vi "tb_host transfer.vi"() -> ()   [LabVIEW 2012]
uses:
  <userlib>/FPGA Library/Code Development/DRAM/2 Bank DRAM/Data Type (256).ctl
  <vilib>/Platform/TimedLoop/XDataNode/timing_clust.ctl
  <vilib>/Platform/TimedLoop/XDataNode/nitl_modes.ctl
  <vilib>/Platform/TimedLoop/XDataNode/wakeup.ctl
  <vilib>/rvi/Emulation/niFpgaSctlEmulationRegisterWithScheduler.vi
  <vilib>/rvi/Emulation/niFpgaSctlEmulationScheduler.vi
  <vilib>/platform/TimedLoop/XDataNode/XDataNode.xnode
  <vilib>/Platform/TimedLoop/XDataNode/XDNodeRunTimeDep.lvlib
panel:
  in  "stop":bool
  out "Data into FIFO":u64[](array[numeric])
  out "Input Data":T1
  out "Data to FIFO":u64(graph)
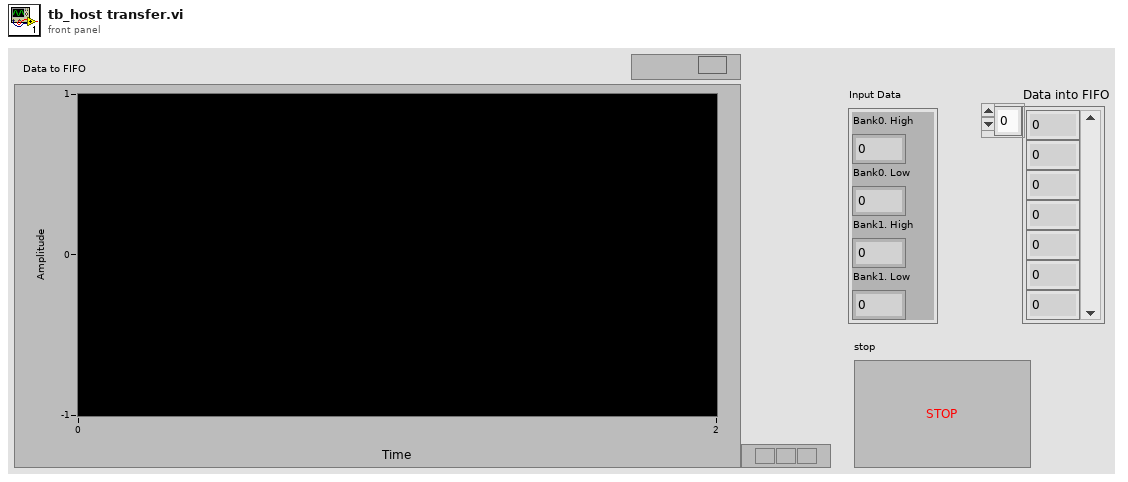
[diagram p1: front panel]
types:
  T1 = typedef "Data Type (256).ctl" = cluster{"Bank0. High":u64, "Bank0. Low":u64, "Bank1. High":u64, "Bank1. Low":u64}
  T2 = typedef "XDNodeRunTimeDep.lvlib/timing_clust.ctl" = cluster{"Expected End [f-1]":u64, "Actual End [f-1]":u64, "Finished Late? [f-1]":bool, "Expected End [i-1]":u64, "Actual End [i-1]":u64, "Finished Late? [i-1]":bool, "Expected Start [i]":u64, "Actual Start [i]":u64, "Expected Start [f]":u64, "Actual Start [f]":u64, "Source Name":string, "Structure Name":string, "Period":i64, "Deadline":i64, "Offset":i64, "Start":i64, "Priority":i32, "Timeout":i32, "Mode":T3, "Wakeup Reason":T4, "Error":errorcluster, "Source Type":string, "Secondary Source Type":string, "Global End Time":u64, "Global Start Time":u64, "Frame Duration":u64, "Iteration Duration":u64, "Assigned CPU":i32, "I/O Scan Engine Mode":u32}
  T3 = typedef "XDNodeRunTimeDep.lvlib/nitl_modes.ctl" = enum32{"No Change", "Process missed periods, maintain original phase", "Discard missed periods, maintain original phase", "Process missed periods, ignore original phase", "Discard missed periods, ignore original phase"}
  T4 = typedef "XDNodeRunTimeDep.lvlib/wakeup.ctl" = enum32{"Normal", "Aborted", "Asynchronous wakeup", "Timing source error", "Timed loop error", "Timeout"}
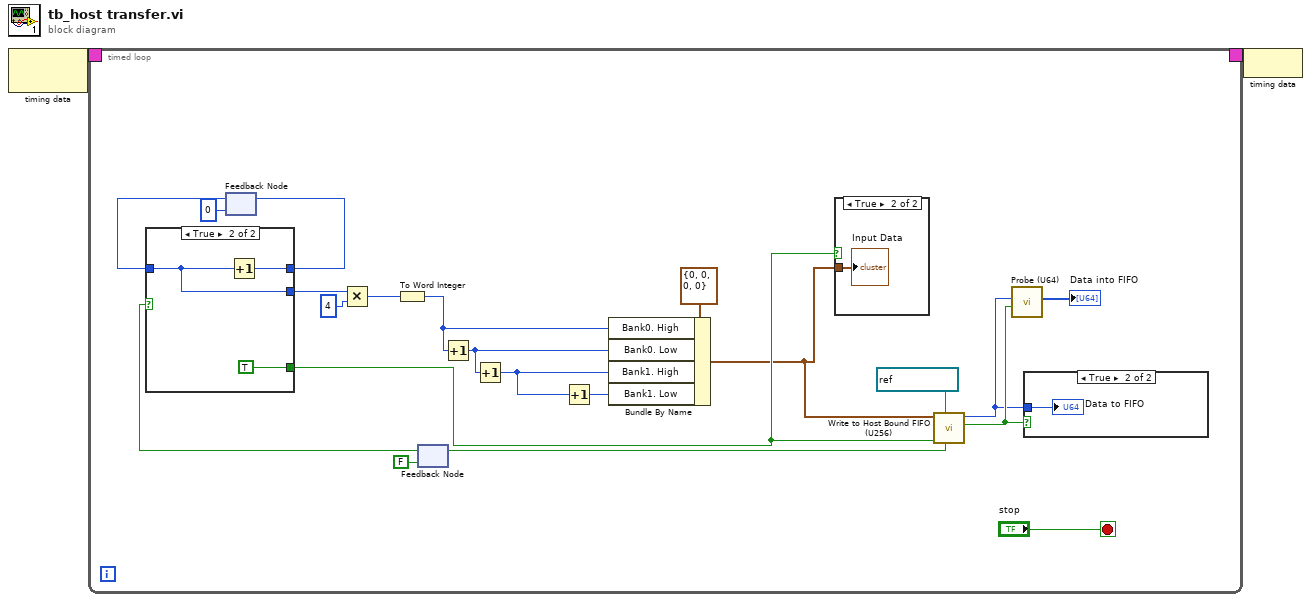
[diagram p0: block diagram]
diagram:
  n1 = node-c288() -> (w2:T2)  [unwired: 1 in]
  n2 = timed-loop {
    timing: w2 -> [_]
    timing-out: [_] -> w1
    stop <- "stop" stop-if-true
    n3 = feedback #1(u32 0) -> (w13:u32)
    n4 = feedback #2(FALSE ("Ready For Input")) -> (w14:bool)
    n5 = case shown="True" w14 {
      tunnel: w13 -> [w25 w26]
      tunnel: [w25 w28] -> w11
      tunnel: [_ TRUE] -> w10
      tunnel: [w25 w26] -> w8
      frame False {
      }
      frame True {
        n6 = Increment(x=w26) -> (x+1=w28:u32)
      }
    }
    n7 = feedback-in #1(w11) -> ()
    n8 = Multiply(x=w8, y=u32 4) -> (x*y=w21:u32)
    n9 = To Word Integer(number=w21) -> (16bit integer=w20:i16)
    n10 = Increment(x=w20) -> (x+1=w17:i16)
    n11 = Increment(x=w17) -> (x+1=w18:i16)
    n12 = Increment(x=w18) -> (x+1=w19:i16)
    n13 = Bundle By Name(cluster=T1 {"Bank0. High"=0, "Bank0. Low"=0, "Bank1. High"=0, "Bank1. Low"=0} ("Input Data"), "Bank0. High"=w20, "Bank0. Low"=w17, "Bank1. High"=w18, "Bank1. Low"=w19) -> (w9:T1)
    n14 = case shown="True" w10 {
      tunnel: w9 -> [_ w24]
      frame False {
      }
      frame True {
        "Input Data" <- w24
      }
    }
    n15 = call <userlib>:"Write to Host Bound FIFO (U256).vi"("Host FIFO"=refnum<k21> "To Host", "Input Valid"=w10, "Input Data"=w9) -> ("Data Written"=w5:bool, "data out"=w4:u64, "Ready For Input"=w16:bool)  [unwired: 6 in]
    n16 = feedback-in #2(w16) -> ()
    n17 = call <userlib>:"Probe (U64).vi"("Data Valid"=w5, "Input Data"=w4) -> ("Collected Data"=→"Data into FIFO":u64[])  [unwired: 9 in]
    n18 = case shown="True" w5 {
      tunnel: w4 -> [_ w29]
      frame False {
      }
      frame True {
        "Data to FIFO" <- w29
      }
    }
  }
  n19 = node-c288(w1) -> ()
